vi "Run Thermal Models.vi"(7 "thermal dt":dbl, 8 "Error In":errorcluster, 10 "CD state in":T1[](array[typedef]), 11 "ambient T, sensor t0, and heat params":dbl[](array[numeric])) -> (0 "Error Out":errorcluster, 2 "CD  state out":T1[](array[typedef]))   [LabVIEW 2014, in "UEGO Sim Engine.lvlib"]
uses:
  UEGO Sim Engine.lvlib
  UEGO CD state.ctl
  Shared/UEGO fpga inputs.ctl
  Shared/UEGO fpga outputs.ctl
  Shared/VS input channels.ctl
  Shared/VS output channels.ctl
  <vilib>/NI Veristand/Custom Device Tools/Custom Device Utility Library/Custom Device Utility Library.lvlib
  Shared/UEGO Sim Shared.lvlib
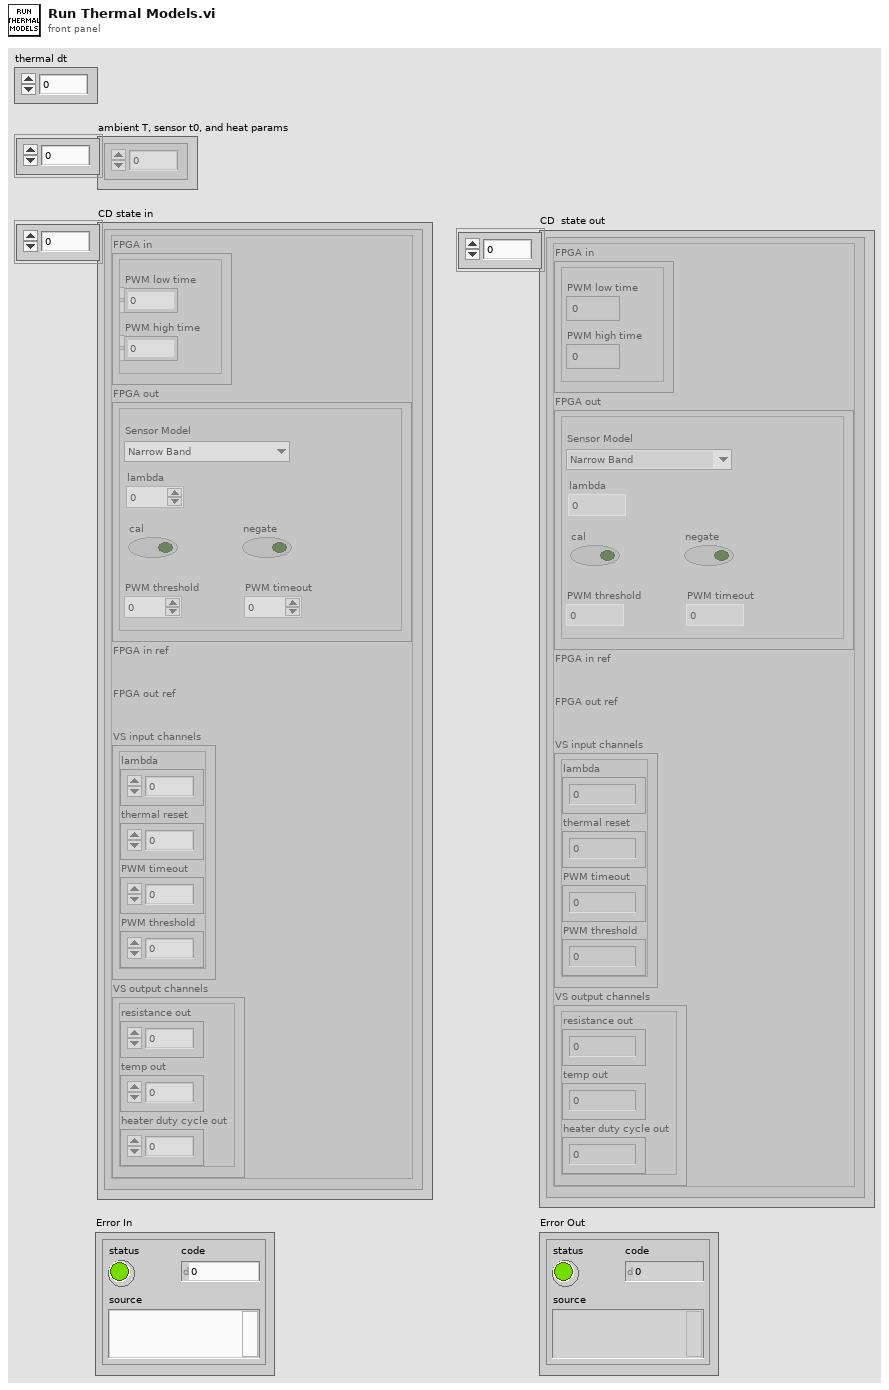
[diagram p1: front panel]
types:
  T1 = typedef "UEGO Sim Engine.lvlib/UEGO CD state.ctl" = cluster{"FPGA in":T2, "FPGA out":T3, "FPGA in ref":refnum<k20>, "FPGA out ref":refnum<k20>, "VS input channels":T5, "VS output channels":T6}
  T2 = typedef "UEGO Sim Shared.lvlib/UEGO fpga inputs.ctl" = cluster{"PWM low time":u32, "PWM high time":u32}
  T3 = typedef "UEGO Sim Shared.lvlib/UEGO fpga outputs.ctl" = cluster{"Sensor Model":T4, "lambda":fxp<+,12,3>, "cal":bool, "negate":bool, "PWM threshold":i16, "PWM timeout":u32}
  T4 = typedef "UEGO Sim Shared.lvlib/sensor models" = enum16{"Narrow Band", "Bosch 4.2", "Bosch 4.9"}
  T5 = typedef "UEGO Sim Shared.lvlib/VS input channels.ctl" = cluster{"lambda":dbl, "thermal reset":dbl, "PWM timeout":dbl, "PWM threshold":dbl}
  T6 = typedef "UEGO Sim Shared.lvlib/VS output channels.ctl" = cluster{"resistance out":dbl, "temp out":dbl, "heater duty cycle out":dbl}
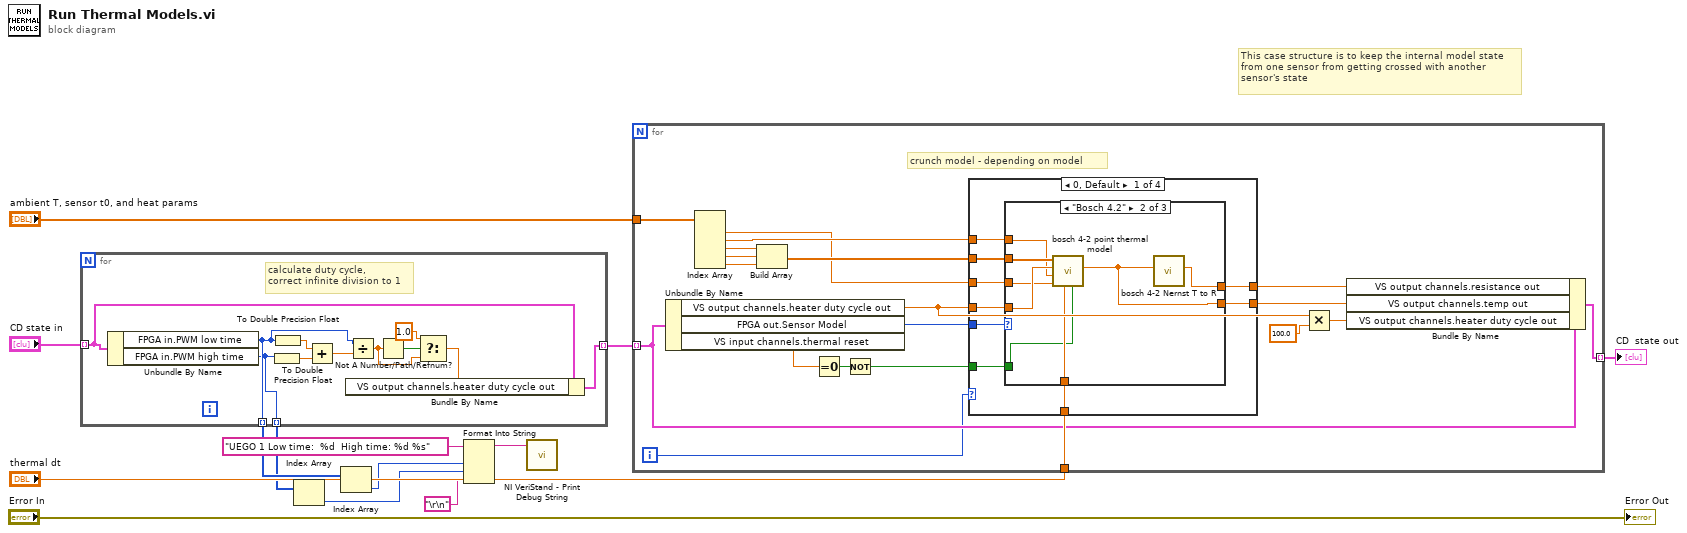
[diagram p0: block diagram]
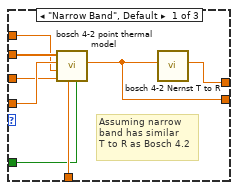
[diagram p2: hidden frame]
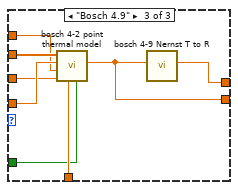
[diagram p3: hidden frame]
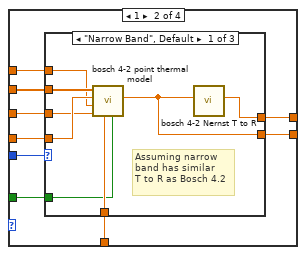
[diagram p4: hidden frame]
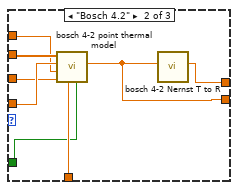
[diagram p5: hidden frame]
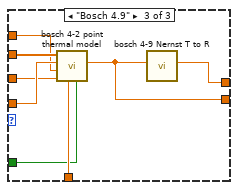
[diagram p6: hidden frame]
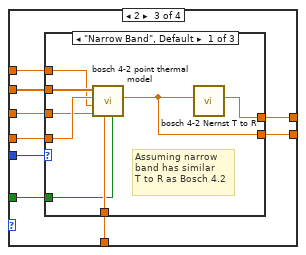
[diagram p7: hidden frame]
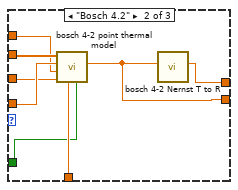
[diagram p8: hidden frame]
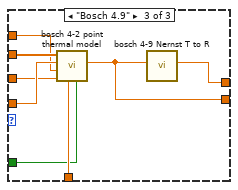
[diagram p9: hidden frame]
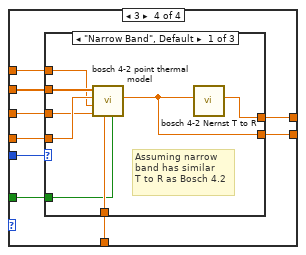
[diagram p10: hidden frame]
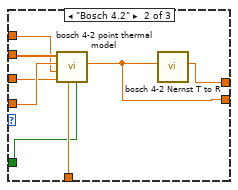
[diagram p11: hidden frame]
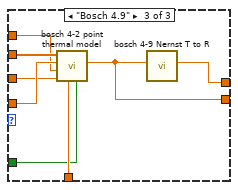
[diagram p12: hidden frame]
diagram:
  # "This case structure is to keep the internal model state\nfrom one sensor from getting crossed with another\nsensor's state"
  n1 = for {
    tunnel: "CD state in" -> [w18] mode=indexing
    tunnel: [w16] -> w9 mode=indexing
    tunnel: [w15] -> w7 mode=indexing
    tunnel: [w14] -> w6 mode=indexing
    # "calculate duty cycle, \ncorrect infinite division to 1"
    n2 = Unbundle By Name(w18) -> ("FPGA in.PWM low time"=w15:u32, "FPGA in.PWM high time"=w14:u32)
    n3 = To Double Precision Float(number=w14) -> (double precision float=w24:dbl)
    n4 = To Double Precision Float(number=w15) -> (double precision float=w23:dbl)
    n5 = Add(x=w23, y=w24) -> (x+y=w22:dbl)
    n6 = Divide(x=w15, y=w22) -> (x/y=w20:dbl)
    n7 = Not A Number/Path/Refnum?(number/path/refnum=w20) -> (NaN/Path/Refnum?=w21:bool)
    n8 = Select(t=1.0, s=w21, f=w20) -> (s? t:f=w17:dbl)
    n9 = Bundle By Name(cluster=w18, "VS output channels.heater duty cycle out"=w17) -> (w16:T1)
  }
  n10 = Index Array(array=w6) -> (element=w3:u32)  [unwired: 1 in]
  n11 = Index Array(array=w7) -> (element=w5:u32)  [unwired: 1 in]
  n12 = Format Into String(format string="UEGO 1 Low time:  %d  High time: %d %s", w5, w3, "\r\n") -> (resulting string=w1:string)  [unwired: 2 in, 1 out]
  n13 = call <vilib>:"NI VeriStand - Print Debug String.vi"("Message"=w1) -> ()  [unwired: 10 in, 1 out]
  n14 = for {
    tunnel: "ambient T, sensor t0, and heat params" -> [w43]
    tunnel: [w32] -> w8 mode=indexing
    tunnel: "thermal dt" -> [w36]
    tunnel: w9 -> [w29] mode=indexing
    i -> [w28]
    # "crunch model - depending on model"
    n15 = Unbundle By Name(w29) -> ("VS output channels.heater duty cycle out"=w26:dbl, "FPGA out.Sensor Model"=w44:T4, "VS input channels.thermal reset"=w35:dbl)
    n16 = Index Array(array=w43) -> (element #1=w37:dbl, element #2=w38:dbl, element #3=w42:dbl, element #4=w41:dbl, element #5=w40:dbl)  [unwired: 5 in]
    n17 = Build Array(w42, w41, w40) -> (w39:dbl[])
    n18 = Equal To 0?(x=w35) -> (x = 0?=w34:bool)
    n19 = Not(x=w34) -> (.not. x?=w33:bool)
    n20 = case shown="0, Default" w28 {
      tunnel: w44 -> [w53 w86 w119 w152]
      tunnel: w39 -> [w52 w85 w118 w151]
      tunnel: w26 -> [w51 w84 w117 w150]
      tunnel: w38 -> [w50 w83 w116 w149]
      tunnel: w37 -> [w49 w82 w115 w148]
      tunnel: w36 -> [w48 w81 w114 w147]
      tunnel: w33 -> [w47 w80 w113 w146]
      tunnel: [w46 w79 w112 w145] -> w31
      tunnel: [w45 w78 w111 w144] -> w30
      frame 0, Default {
        n21 = case shown="\"Bosch 4.2\"" w53 {
          tunnel: w52 -> [w57 w63 w77]
          tunnel: w51 -> [w59 w65 w76]
          tunnel: w50 -> [w56 w62 w75]
          tunnel: w49 -> [w58 w64 w74]
          tunnel: w48 -> [w61 w67 w73]
          tunnel: w47 -> [w60 w66 w72]
          tunnel: [w55 w69 w71] -> w46
          tunnel: [w54 w68 w70] -> w45
          frame "Narrow Band", Default {
            # "Assuming narrow\nband has similar\nT to R as Bosch 4.2"
            n22 = call "bosch 4-2 point thermal model.vi"("Reset?"=w60, "dt"=w61, "Ambient Temp"=w58, "Sensor T0"=w56, "Duty Cycle %"=w59, "X"=w57) -> ("T"=w55:dbl)  [unwired: 5 in]
            n23 = call "bosch 4-2 Nernst T to R.vi"("Temperature (C)"=w55) -> ("Resistance (Ohms)"=w54:dbl)  [unwired: 10 in]
          }
          frame "Bosch 4.2" {
            n24 = call "bosch 4-2 point thermal model.vi"("Reset?"=w66, "dt"=w67, "Ambient Temp"=w64, "Sensor T0"=w62, "Duty Cycle %"=w65, "X"=w63) -> ("T"=w69:dbl)  [unwired: 5 in]
            n25 = call "bosch 4-2 Nernst T to R.vi"("Temperature (C)"=w69) -> ("Resistance (Ohms)"=w68:dbl)  [unwired: 10 in]
          }
          frame "Bosch 4.9" {
            n26 = call "bosch 4-2 point thermal model.vi"("Reset?"=w72, "dt"=w73, "Ambient Temp"=w74, "Sensor T0"=w75, "Duty Cycle %"=w76, "X"=w77) -> ("T"=w71:dbl)  [unwired: 5 in]
            n27 = call "bosch 4-9 Nernst T to R.vi"("T"=w71) -> ("R"=w70:dbl)  [unwired: 10 in]
          }
        }
      }
      frame 1 {
        n28 = case shown="\"Narrow Band\", Default" w86 {
          tunnel: w85 -> [w90 w96 w110]
          tunnel: w84 -> [w92 w98 w109]
          tunnel: w83 -> [w89 w95 w108]
          tunnel: w82 -> [w91 w97 w107]
          tunnel: w81 -> [w94 w100 w106]
          tunnel: w80 -> [w93 w99 w105]
          tunnel: [w88 w102 w104] -> w79
          tunnel: [w87 w101 w103] -> w78
          frame "Narrow Band", Default {
            # "Assuming narrow\nband has similar\nT to R as Bosch 4.2"
            n29 = call "bosch 4-2 point thermal model.vi"("Reset?"=w93, "dt"=w94, "Ambient Temp"=w91, "Sensor T0"=w89, "Duty Cycle %"=w92, "X"=w90) -> ("T"=w88:dbl)  [unwired: 5 in]
            n30 = call "bosch 4-2 Nernst T to R.vi"("Temperature (C)"=w88) -> ("Resistance (Ohms)"=w87:dbl)  [unwired: 10 in]
          }
          frame "Bosch 4.2" {
            n31 = call "bosch 4-2 point thermal model.vi"("Reset?"=w99, "dt"=w100, "Ambient Temp"=w97, "Sensor T0"=w95, "Duty Cycle %"=w98, "X"=w96) -> ("T"=w102:dbl)  [unwired: 5 in]
            n32 = call "bosch 4-2 Nernst T to R.vi"("Temperature (C)"=w102) -> ("Resistance (Ohms)"=w101:dbl)  [unwired: 10 in]
          }
          frame "Bosch 4.9" {
            n33 = call "bosch 4-2 point thermal model.vi"("Reset?"=w105, "dt"=w106, "Ambient Temp"=w107, "Sensor T0"=w108, "Duty Cycle %"=w109, "X"=w110) -> ("T"=w104:dbl)  [unwired: 5 in]
            n34 = call "bosch 4-9 Nernst T to R.vi"("T"=w104) -> ("R"=w103:dbl)  [unwired: 10 in]
          }
        }
      }
      frame 2 {
        n35 = case shown="\"Narrow Band\", Default" w119 {
          tunnel: w118 -> [w123 w129 w143]
          tunnel: w117 -> [w125 w131 w142]
          tunnel: w116 -> [w122 w128 w141]
          tunnel: w115 -> [w124 w130 w140]
          tunnel: w114 -> [w127 w133 w139]
          tunnel: w113 -> [w126 w132 w138]
          tunnel: [w121 w135 w137] -> w112
          tunnel: [w120 w134 w136] -> w111
          frame "Narrow Band", Default {
            # "Assuming narrow\nband has similar\nT to R as Bosch 4.2"
            n36 = call "bosch 4-2 point thermal model.vi"("Reset?"=w126, "dt"=w127, "Ambient Temp"=w124, "Sensor T0"=w122, "Duty Cycle %"=w125, "X"=w123) -> ("T"=w121:dbl)  [unwired: 5 in]
            n37 = call "bosch 4-2 Nernst T to R.vi"("Temperature (C)"=w121) -> ("Resistance (Ohms)"=w120:dbl)  [unwired: 10 in]
          }
          frame "Bosch 4.2" {
            n38 = call "bosch 4-2 point thermal model.vi"("Reset?"=w132, "dt"=w133, "Ambient Temp"=w130, "Sensor T0"=w128, "Duty Cycle %"=w131, "X"=w129) -> ("T"=w135:dbl)  [unwired: 5 in]
            n39 = call "bosch 4-2 Nernst T to R.vi"("Temperature (C)"=w135) -> ("Resistance (Ohms)"=w134:dbl)  [unwired: 10 in]
          }
          frame "Bosch 4.9" {
            n40 = call "bosch 4-2 point thermal model.vi"("Reset?"=w138, "dt"=w139, "Ambient Temp"=w140, "Sensor T0"=w141, "Duty Cycle %"=w142, "X"=w143) -> ("T"=w137:dbl)  [unwired: 5 in]
            n41 = call "bosch 4-9 Nernst T to R.vi"("T"=w137) -> ("R"=w136:dbl)  [unwired: 10 in]
          }
        }
      }
      frame 3 {
        n42 = case shown="\"Narrow Band\", Default" w152 {
          tunnel: w151 -> [w156 w162 w176]
          tunnel: w150 -> [w158 w164 w175]
          tunnel: w149 -> [w155 w161 w174]
          tunnel: w148 -> [w157 w163 w173]
          tunnel: w147 -> [w160 w166 w172]
          tunnel: w146 -> [w159 w165 w171]
          tunnel: [w154 w168 w170] -> w145
          tunnel: [w153 w167 w169] -> w144
          frame "Narrow Band", Default {
            # "Assuming narrow\nband has similar\nT to R as Bosch 4.2"
            n43 = call "bosch 4-2 point thermal model.vi"("Reset?"=w159, "dt"=w160, "Ambient Temp"=w157, "Sensor T0"=w155, "Duty Cycle %"=w158, "X"=w156) -> ("T"=w154:dbl)  [unwired: 5 in]
            n44 = call "bosch 4-2 Nernst T to R.vi"("Temperature (C)"=w154) -> ("Resistance (Ohms)"=w153:dbl)  [unwired: 10 in]
          }
          frame "Bosch 4.2" {
            n45 = call "bosch 4-2 point thermal model.vi"("Reset?"=w165, "dt"=w166, "Ambient Temp"=w163, "Sensor T0"=w161, "Duty Cycle %"=w164, "X"=w162) -> ("T"=w168:dbl)  [unwired: 5 in]
            n46 = call "bosch 4-2 Nernst T to R.vi"("Temperature (C)"=w168) -> ("Resistance (Ohms)"=w167:dbl)  [unwired: 10 in]
          }
          frame "Bosch 4.9" {
            n47 = call "bosch 4-2 point thermal model.vi"("Reset?"=w171, "dt"=w172, "Ambient Temp"=w173, "Sensor T0"=w174, "Duty Cycle %"=w175, "X"=w176) -> ("T"=w170:dbl)  [unwired: 5 in]
            n48 = call "bosch 4-9 Nernst T to R.vi"("T"=w170) -> ("R"=w169:dbl)  [unwired: 10 in]
          }
        }
      }
    }
    n49 = Multiply(x=w26, y=100.0) -> (x*y=w27:dbl)
    n50 = Bundle By Name(cluster=w29, "VS output channels.resistance out"=w30, "VS output channels.temp out"=w31, "VS output channels.heater duty cycle out"=w27) -> (w32:T1)
  }
  "CD  state out" <- w8
  "Error Out" <- "Error In"
